vi "add_instrument_interface.vi"(0 "VI Ref In":refnum<vi>, 11 "error in":errorcluster) -> (4 "VI Ref Out":refnum<vi>, 15 "error out":errorcluster)   [LabVIEW 2018]
uses:
  Iternl/CalPos/CmdToStr/TypeDefinitions/main_position_types.ctl
  Misc/AddNode/TypeDefinitions/node_types.ctl
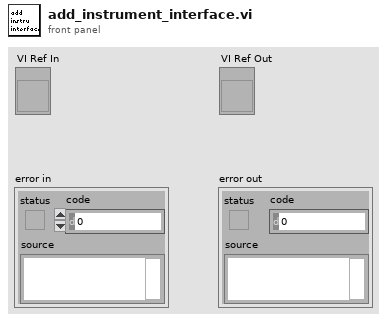
[diagram p1: front panel]
types:
  T1 = typedef "node_types.ctl" = enum16{"FormatIntoString", "PickLine", "AppendTrueFalse", "VISAWrite", "SubVI", "ConcatenateStrings", "VISARead", "ProperyNode", "ScanFromString", "SpreadSheetStringToArray"}
  T2 = typedef "main_position_types.ctl" = enum16{"Node", "FormatNodeForMultipleControls", "BoolConstant", "FormatConstant", "1stSubNodeX"}
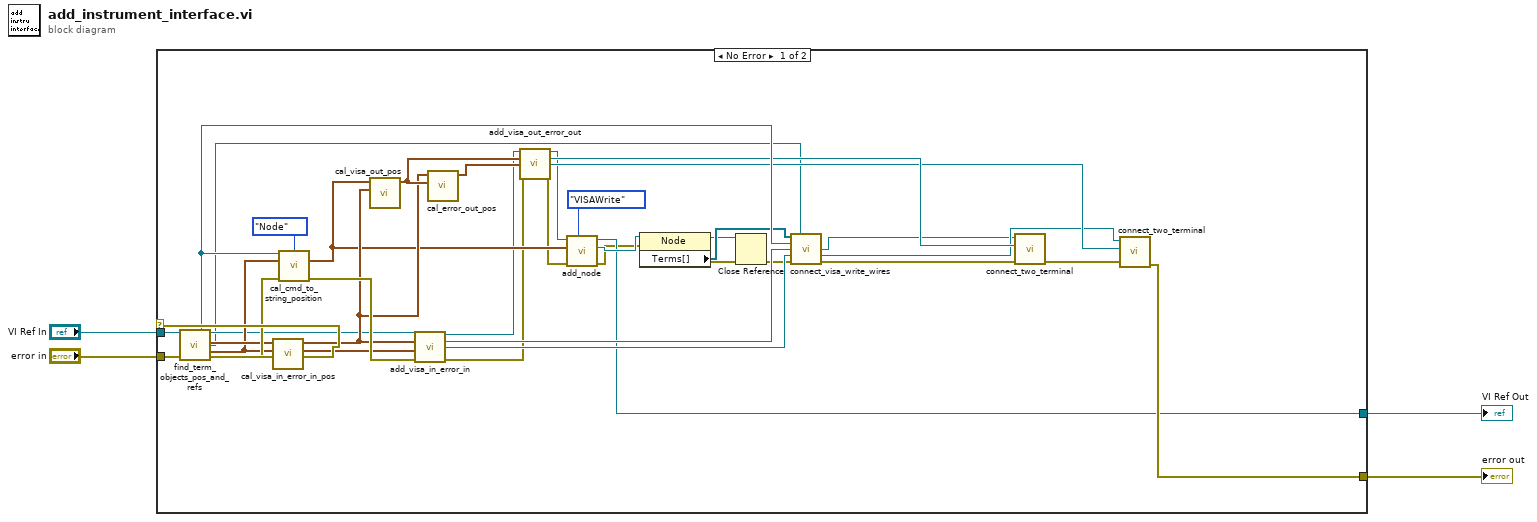
[diagram p0: block diagram]
diagram:
  n1 = case shown="No Error" "error in" {
    tunnel: [w40 w41] -> w4
    tunnel: [w19 w42] -> w3
    tunnel: "VI Ref In" -> [w16 w42]
    tunnel: "error in" -> [w15 w41]
    frame No Error {
      n2 = call "find_term_objects_pos_and_refs.vi"("VI Ref In"=w16, "error in (no error)"=w15) -> ("Last Function"=w31:refnum<vi>, "VI Ref Out"=w13:refnum<vi>, "Last Control Position"=w33:cluster{"Left":i32, "Top":i32}, "Last StrCnst Refnum"=w6:refnum<vi>, "Last Function Position"=w32:cluster{"Left":i32, "Top":i32}, "error out"=w37:errorcluster)  [unwired: 8 out]
      n3 = call "cal_visa_in_error_in_pos.vi"("Last Function Position"=w32, "Last Control Position"=w33) -> ("Error In Position"=w14:cluster{"Left":i32, "Top":i32}, "Visa In Position"=w35:cluster{"Left":i32, "Top":i32})  [unwired: 8 out]
      n4 = call "cal_cmd_to_string_position.vi"("Last Function Ref In"=w31, "Enum"=main_position_types."Node", "Main Node BD Position"=w32, "error in (no error)"=w37) -> ("Main Node Position/Enable Constant Position"=w34:cluster{"Left":u32, "Top":i32}, "error out"=w38:errorcluster)  [unwired: 3 in, 7 out]
      n5 = call "cal_visa_out_pos.vi"("Visa In Position"=w35, "Main Node Position"=w34) -> ("Visa Out  Position"=w36:cluster{"Left":u32, "Top":i32})  [unwired: 2 in, 7 out]
      n6 = call "add_visa_in_error_in.vi"("VI Ref In"=w13, "Visa In Position"=w35, "Error In Position"=w14, "error in"=w38) -> ("VI Ref Out"=w10:refnum<vi>, "VISA In Term"=w24:refnum<vi>, "Error In Term"=w25:refnum<vi>, "error out"=w9:errorcluster)  [unwired: 1 in, 7 out]
      n7 = call "cal_error_out_pos.vi"("Visa Out  Position"=w36, "Last Function Position"=w35) -> ("Error Out  Position"=w18:cluster{"Left":u32, "Top":i32})  [unwired: 9 out]
      n8 = call "add_visa_out_error_out.vi"("VI Ref In"=w10, "Visa Out  Position"=w36, "Error Out  Position"=w18, "error in"=w9) -> ("VI Ref Out"=w11:refnum<vi>, "Visa Out Term"=w29:refnum<vi>, "Error Out Term"=w28:refnum<vi>, "error out"=w8:errorcluster)  [unwired: 8 out]
      n9 = call "add_node.vi"("Node Type"=node_types."VISAWrite", "error in (no error)"=w8, "BD Position"=w34, "VI Ref In"=w11) -> ("error out"=w12:errorcluster, "Node Refnum"=w20:refnum<vi>, "VI Ref Out"=w19:refnum<vi>)  [unwired: 2 in, 3 out]
      n10 = property class="Node"(reference=w20, error in=w12) -> (reference out=w21:refnum<vi>, error out=w22:errorcluster, "Terms[]"=w30:refnum<vi>[])
      n11 = Close Reference(reference=w21, error in (no error)=w22) -> (error out=w23:errorcluster)
      n12 = call "connect_visa_write_wires.vi"("Terms[]"=w30, "Last StrCnst Refnum"=w6, "Last Function"=w31, "VISA In Term"=w24, "Error In Term"=w25, "error in"=w23) -> ("Visa Out Term"=w26:refnum<vi>, "Error Out Term"=w27:refnum<vi>, "error out"=w7:errorcluster)  [unwired: 1 in, 6 out]
      n13 = call "connect_two_terminal.vi"("error in"=w7, "Terminal 2"=w29, "Terminal 1"=w26) -> ("error out"=w5:errorcluster)  [unwired: 1 in, 7 out]
      n14 = call "connect_two_terminal.vi"("error in"=w5, "Terminal 2"=w28, "Terminal 1"=w27) -> ("error out"=w40:errorcluster)  [unwired: 1 in, 7 out]
    }
    frame Error {
    }
  }
  "error out" <- w4
  "VI Ref Out" <- w3
